vi "target distance and angle.vi"(10 "x side":dbl, 11 "x center":dbl) -> (2 "target angle in degrees":dbl, 3 "distance from target in inches":dbl)   [LabVIEW 2018]
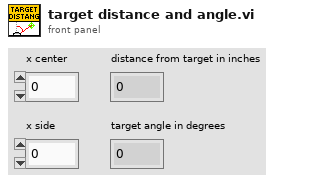
[diagram p1: front panel]
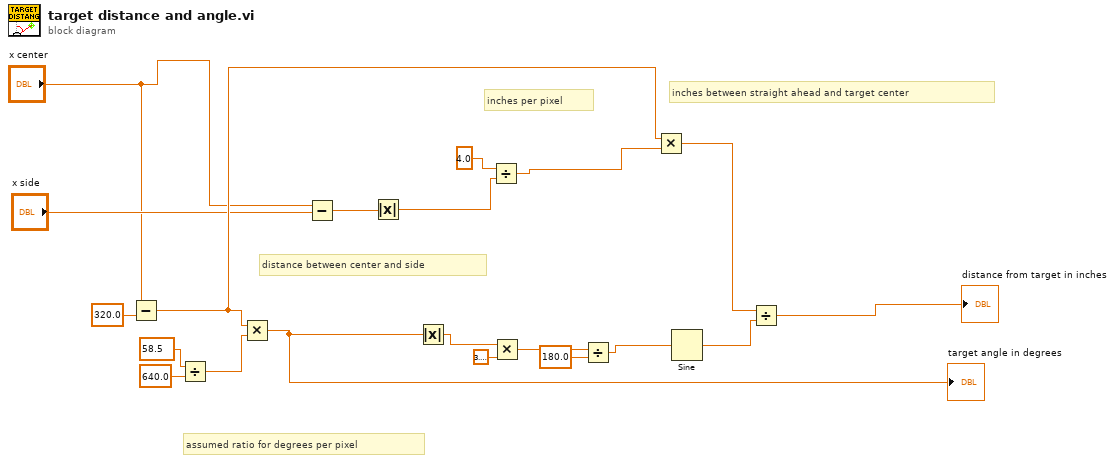
[diagram p0: block diagram]
diagram:
  # "assumed ratio for degrees per pixel"
  # "distance between center and side"
  # "inches between straight ahead and target center"
  # "inches per pixel"
  n1 = Subtract(x="x center", y=320.0) -> (x-y=w20:dbl)
  n2 = Divide(x=58.5, y=640.0) -> (x/y=w7:dbl)
  n3 = Multiply(x=w20, y=w7) -> (x*y=w8:dbl)
  "target angle in degrees" <- w8
  n4 = Subtract(x="x center", y="x side") -> (x-y=w11:dbl)
  n5 = Absolute Value(x=w11) -> (abs(x)=w12:dbl)
  n6 = Absolute Value(x=w8) -> (abs(x)=w13:dbl)
  n7 = Divide(x=4.0, y=w12) -> (x/y=w2:dbl)
  n8 = Multiply(x=w13, y=3.141592653589793) -> (x*y=w16:dbl)
  n9 = Divide(x=w16, y=180.0) -> (x/y=w17:dbl)
  n10 = Multiply(x=w20, y=w2) -> (x*y=w4:dbl)
  n11 = Sine(x=w17) -> (sin(x)=w14:dbl)
  n12 = Divide(x=w4, y=w14) -> (x/y=→"distance from target in inches":dbl)
